vi "Read Id_a.vi"(10 "write string":string="id\r" caption="wlaczona opcja \"codes display\"", 11 "VISA resource name":refnum<visa-resource-name>="COM7") -> (2 "read string":string)   [LabVIEW 2017]
uses:
  <vilib>/Instr/_visa.llb/VISA Configure Serial Port (Instr).vi
panel:
  # "wlaczona opcja \"codes display\""
  # "wlaczona opcja \"codes display\""
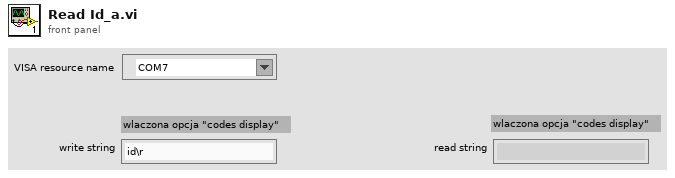
[diagram p1: front panel]
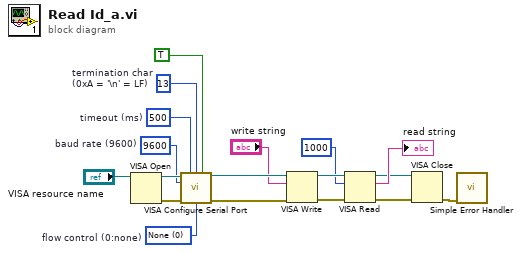
[diagram p0: block diagram]
diagram:
  w11 = u32 9600  # baud rate (9600)
  w12 = u16 0 items=["None", "XON/XOFF", "RTS/CTS", "XON/XOFF & RTS/CTS", "DTR/DSR", "XON/XOFF & DTR/DSR"]  # flow control (0:none)
  w14 = u8 13  # termination char (0xA = '\n' = LF)
  w15 = u32 500  # timeout (ms)
  n1 = VISA Open(VISA resource name="VISA resource name") -> (VISA resource name=w17:refnum<visa-resource-name>, error out=w16:errorcluster)  [unwired: 4 in]
  n2 = call-poly "VISA Configure Serial Port"("VISA resource name"=w17, "timeout (10sec)"=w15, "termination char\n(0xA = '\\n' = LF)"=w14, "Enable Termination\nChar (T)"=TRUE ("Enable Termination\nChar (T)"), "baud rate (9600)"=w11, "error in (no error)"=w16, "flow control (0:none)"=w12) -> ("VISA resource name out"=w9:refnum<visa-resource-name>, "error out"=w10:errorcluster)  [unwired: 7 in]
  n3 = VISA Write(VISA resource name=w9, write buffer="write string", error in (no error)=w10) -> (VISA resource name out=w7:refnum<visa-resource-name>, error out=w8:errorcluster)  [unwired: 1 out]
  n4 = VISA Read(VISA resource name=w7, byte count=u32 1000, error in (no error)=w8) -> (VISA resource name out=w2:refnum<visa-resource-name>, read buffer=→"read string":string, error out=w3:errorcluster)  [unwired: 1 out]
  n5 = VISA Close(VISA resource name=w2, error in (no error)=w3) -> (error out=w1:errorcluster)
  n6 = call <vilib>:"Simple Error Handler.vi"("error in (no error)"=w1) -> ()  [unwired: 4 in, 5 out]
